vi "Get Property Type.vi"(8 "error in":errorcluster, 11 "Property Node":refnum<k20>) -> (0 "error out":errorcluster, 2 "Property Type":T1, 3 "Property Type Node":refnum<k20>)   [LabVIEW 2024, in "Config File Parser.lvlib" / "Property.lvclass"]
uses:
  Property.lvclass
  Property.lvclass/Property.ctl
  <vilib>/xml/NI_XML.lvlib
  <resource>/objmgr/DOMUserDefRef.rc
  Property Type.ctl
  <vilib>/xml/Close Reference(Node).vi
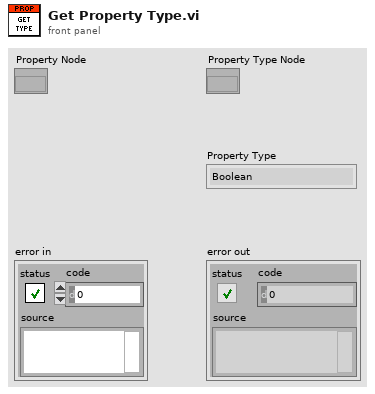
[diagram p1: front panel]
types:
  T1 = typedef "Config File Parser.lvlib/Property.lvclass/Property Type.ctl" = enum16{"Boolean", "Double", "String", "Path", "Dictionary", "DependentFile", "I16", "I32", "I64", "U16", "U32", "U64", "BooleanArray", "DoubleArray", "StringArray", "I16Array", "I32Array", "I64Array", "U16Array", "U32Array", "U64Array"}
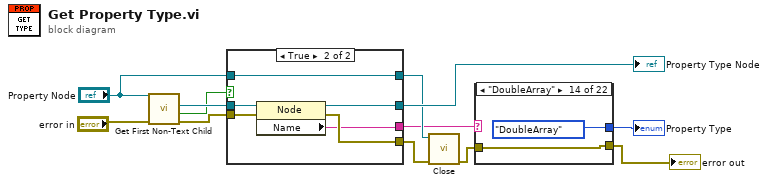
[diagram p0: block diagram]
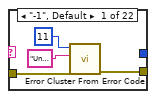
[diagram p2: hidden frame]
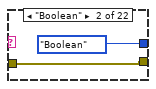
[diagram p3: hidden frame]
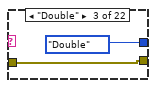
[diagram p4: hidden frame]
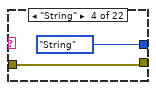
[diagram p5: hidden frame]
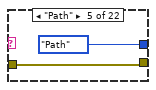
[diagram p6: hidden frame]
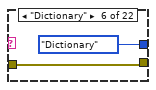
[diagram p7: hidden frame]
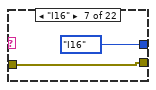
[diagram p8: hidden frame]
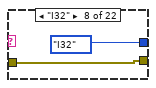
[diagram p9: hidden frame]
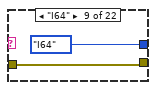
[diagram p10: hidden frame]
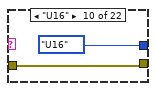
[diagram p11: hidden frame]
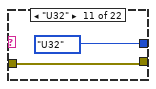
[diagram p12: hidden frame]
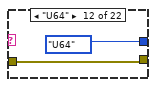
[diagram p13: hidden frame]
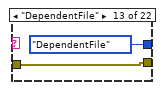
[diagram p14: hidden frame]
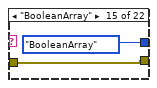
[diagram p15: hidden frame]
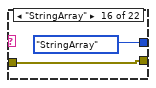
[diagram p16: hidden frame]
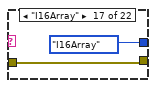
[diagram p17: hidden frame]
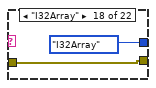
[diagram p18: hidden frame]
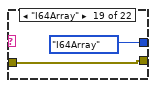
[diagram p19: hidden frame]
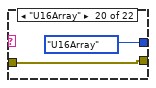
[diagram p20: hidden frame]
diagram:
  n1 = call <vilib>:"Get First Non-Text Child.vi"("error in (no error)"="error in", "node in"="Property Node") -> ("error out"=w11:errorcluster, "found child node?"=w5:bool, "child node"=w7:refnum<k20>)  [unwired: 6 in, 1 out]
  n2 = case shown="True" w5 {
    tunnel: w7 -> [_ w20]
    tunnel: [_ w19] -> w6
    tunnel: w11 -> [w16 w22]
    tunnel: [w15 w21] -> w10
    tunnel: [_ w18] -> w2
    tunnel: [_ w17] -> w3
    tunnel: "Property Node" -> [_ w17]
    frame False {
      n3 = call <vilib>:"Error Cluster From Error Code.vi"("error in (no error)"=w16, "error message (\"\")"="Property should have a \"Type\" attribute", "error code (0)"=10002) -> ("error out"=w15:errorcluster)  [unwired: 6 in]
    }
    frame True {
      n4 = property class="Node"(reference=w20, error in=w22) -> (reference out=w19:refnum<k20>, error out=w21:errorcluster, "Name"=w18:string)
    }
  }
  "Property Type Node" <- w6
  n5 = call-poly <vilib>:"Close.vi"("error in (no error)"=w10, "node"=w3) -> ("error out"=w9:errorcluster)  [unwired: 7 in]
  n6 = case shown="\"DoubleArray\"" w2 {
    tunnel: [_ Property_Type."Boolean" ("Type") Property_Type."Double" ("Type") Property_Type."String" ("Type") Property_Type."Path" ("Type") Property_Type."Dictionary" ("Type") Property_Type."I16" ("Type") Property_Type."I32" ("Type") Property_Type."I64" ("Type") Property_Type."U16" ("Type") Property_Type."U32" ("Type") Property_Type."U64" ("Type") Property_Type."DependentFile" ("Type") Property_Type."DoubleArray" ("Type") Property_Type."BooleanArray" ("Type") Property_Type."StringArray" ("Type") Property_Type."I16Array" ("Type") Property_Type."I32Array" ("Type") Property_Type."I64Array" ("Type") Property_Type."U16Array" ("Type") Property_Type."U32Array" ("Type") Property_Type."U64Array" ("Type")] -> w1
    tunnel: w9 -> [w26 w28 w30 w32 w34 w36 w38 w40 w42 w44 w46 w48 w50 w51 w53 w55 w57 w59 w61 w63 w65 w67]
    tunnel: [w25 w28 w30 w32 w34 w36 w38 w40 w42 w44 w46 w48 w50 w51 w53 w55 w57 w59 w61 w63 w65 w67] -> w8
    frame "-1", Default {
      n7 = call <vilib>:"Error Cluster From Error Code.vi"("error in (no error)"=w26, "error message (\"\")"="UnSupported Property Types are present in the Config File", "error code (0)"=11) -> ("error out"=w25:errorcluster)  [unwired: 6 in]
    }
    frame "Boolean" {
    }
    frame "Double" {
    }
    frame "String" {
    }
    frame "Path" {
    }
    frame "Dictionary" {
    }
    frame "I16" {
    }
    frame "I32" {
    }
    frame "I64" {
    }
    frame "U16" {
    }
    frame "U32" {
    }
    frame "U64" {
    }
    frame "DependentFile" {
    }
    frame "DoubleArray" {
    }
    frame "BooleanArray" {
    }
    frame "StringArray" {
    }
    frame "I16Array" {
    }
    frame "I32Array" {
    }
    frame "I64Array" {
    }
    frame "U16Array" {
    }
    frame "U32Array" {
    }
    frame "U64Array" {
    }
  }
  "Property Type" <- w1
  "error out" <- w8
